vi "Pause.vi"(8 "error in (no error)":errorcluster, 10 "Internal?":bool, 11 "Julabo FP-50 Settings In":T1={"VISA resource name"="", "Simulated?"=FALSE, "Pump Power"=2} {"Pump Power" min=0 max=8 step=1}) -> (0 "error out":errorcluster, 3 "Julabo FP-50 Settings Out":T1={"VISA resource name"="", "Simulated?"=FALSE, "Pump Power"=2} {"Pump Power" min=0 max=8 step=1})   [LabVIEW 2018, in "Julabo Type FP-50 TCU.lvlib"]
uses:
  Julabo Type FP-50 TCU.lvlib
  Julabo FP-50 Settings.ctl
  Third Party Drivers/Julabo Type 1/JULABO DeviceDriver/JULABO DeviceDriver.lvlib
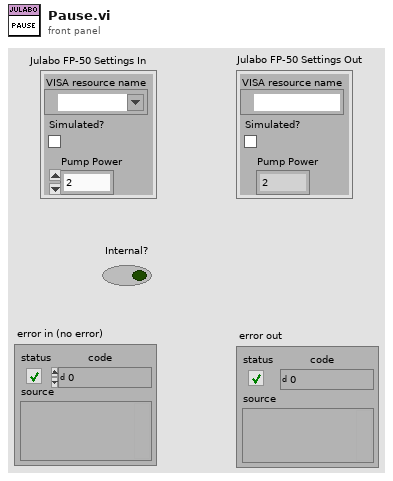
[diagram p1: front panel]
types:
  T1 = typedef "Julabo Type FP-50 TCU.lvlib/Julabo FP-50 Settings.ctl" = cluster{"VISA resource name":refnum<visa-resource-name>, "Simulated?":bool, "Pump Power":i32}
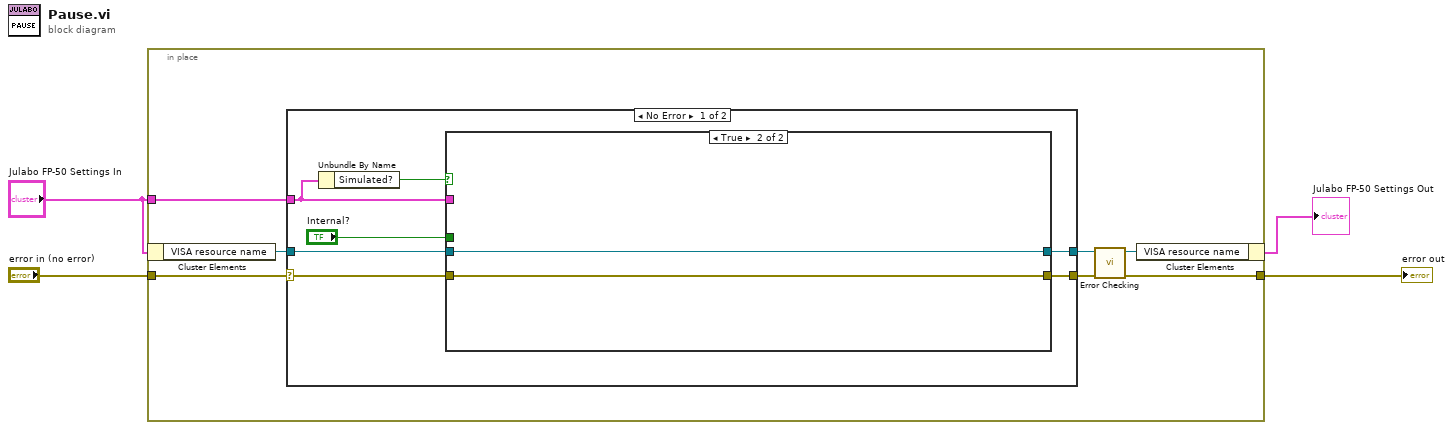
[diagram p0: block diagram]
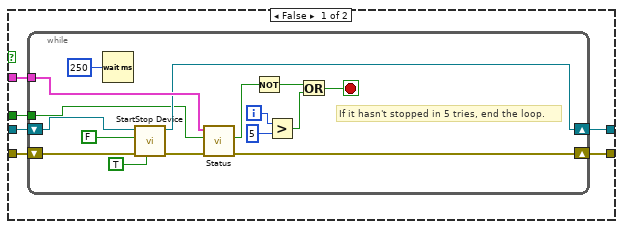
[diagram p2: hidden frame]
diagram:
  n1 = in-place {
    in-place-border: "error in (no error)" -> [w11]
    in-place-border: [w8] -> w3
    in-place-border: "Julabo FP-50 Settings In" -> [w7]
    n2 = in-place-cluster #1("Julabo FP-50 Settings In") -> ("VISA resource name"=w6:refnum<visa-resource-name>)
    n3 = case shown="No Error" w11 {
      selector: w11 -> [w18 w44]
      tunnel: w7 -> [w14 _]
      tunnel: [w17 w44] -> w9
      tunnel: [w16 w43] -> w10
      tunnel: w6 -> [w12 w43]
      frame No Error {
        n4 = Unbundle By Name(w14) -> ("Simulated?"=w15:bool)
        n5 = case shown="True" w15 {
          tunnel: w18 -> [w22 w42]
          tunnel: [w20 w42] -> w17
          tunnel: [w24 w41] -> w16
          tunnel: w12 -> [w23 w41]
          tunnel: w14 -> [w21 _]
          tunnel: "Internal?" -> [w19 _]
          frame False {
            n6 = while {
              tunnel: w21 -> [w40]
              shift-right: [w27] -> w24
              shift-left: w23 -> [w30]
              shift-right: [w39] -> w20
              shift-left: w22 -> [w29]
              tunnel: w19 -> [w26]
              i -> [w37]
              stop <- w38 stop-if-true
              # "If it hasn't stopped in 5 tries, end the loop."
              n7 = Wait (ms)(milliseconds to wait=u32 250) -> ()  [unwired: 1 out]
              n8 = call "StartStop Device.vi"("parseError? T:Yes"=TRUE, "error in (no error)"=w29, "Start/Stop (f:Stop)"=FALSE, "VISA resource name"=w30) -> ("error out"=w28:errorcluster, "VISA resource name out"=w27:refnum<visa-resource-name>)  [unwired: 6 in]
              n9 = call "Status.vi"("error in (no error)"=w28, "Internal?"=w26, "Julabo FP-50 Settings"=w40) -> ("error out"=w39:errorcluster, "Running"=w32:bool)  [unwired: 3 in, 4 out]
              n10 = Not(x=w32) -> (.not. x?=w33:bool)
              n11 = Greater?(x=w37, y=5) -> (0:w35:bool)
              n12 = Or(x=w33, y=w35) -> (x .or. y?=w38:bool)
            }
          }
          frame True {
          }
        }
      }
      frame Error {
      }
    }
    n13 = call "Error Checking.vi"("error in (no error)"=w9, "VISA resource name"=w10) -> ("error out"=w8:errorcluster, "VISA resource name"=w5:refnum<visa-resource-name>)  [unwired: 7 in, 1 out]
    n14 = in-place-cluster #1("VISA resource name"=w5) -> (→"Julabo FP-50 Settings Out":T1)
  }
  "error out" <- w3
